vi "Save Station Information.vi"(8 "error in (no error)":errorcluster, 10 "Station Info":T1, 11 "TestMonitor in":refnum<class "TestMonitor.lvclass">) -> (0 "error out":errorcluster, 3 "TestMonitor out":refnum<class "TestMonitor.lvclass">)   [LabVIEW 2018, in "TestMonitor.lvclass"]
doc: "This VI will save the Station Information to the permanent report."
uses:
  TestMonitor.lvclass
  Report Information/Station Information.ctl
  TestMonitor.lvclass/TestMonitor.ctl
  <vilib>/Skyline/TestMonitor/Test Result/Update Test Result (Single).vi
  <vilib>/Skyline/TestMonitor/Test Result/NI SystemLink Test Result.lvclass
  Report Information/Report Information.lvclass
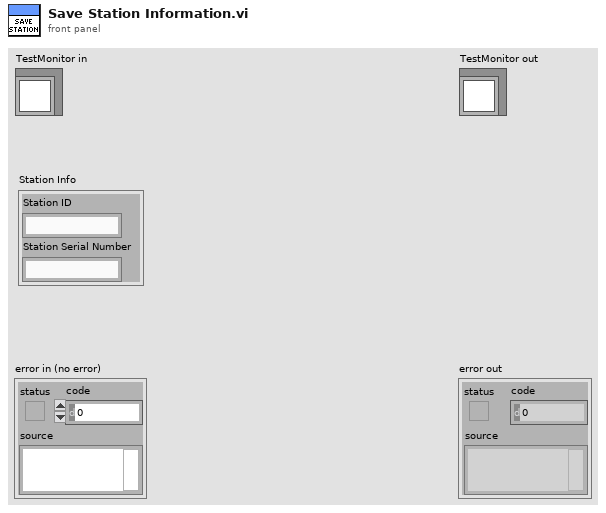
[diagram p1: front panel]
types:
  T1 = typedef "Report Information.lvclass/Station Information.ctl" = cluster{"Station ID":string, "Station Serial Number":string}
  T2 = typedef "NI Skyline Utilities.lvlib/Property.ctl" = cluster{"key":string, "value":string}
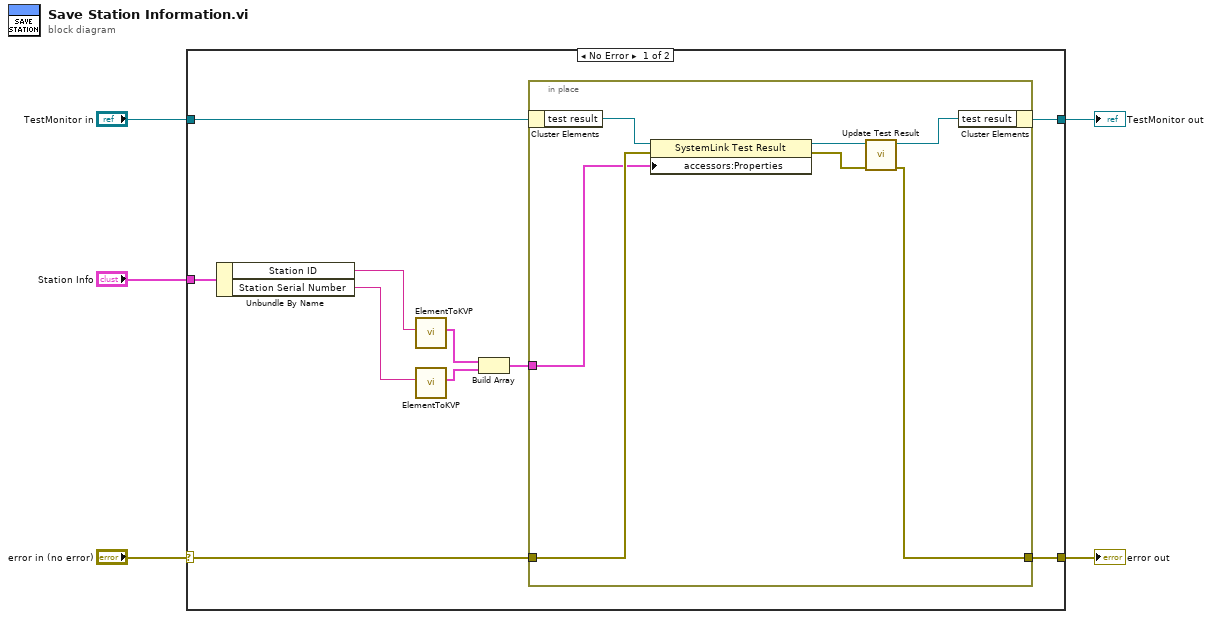
[diagram p0: block diagram]
diagram:
  n1 = case shown="No Error" "error in (no error)" {
    selector: "error in (no error)" -> [w12 w23]
    tunnel: [w10 w23] -> w5
    tunnel: [w14 w24] -> w3
    tunnel: "TestMonitor in" -> [w15 w24]
    tunnel: "Station Info" -> [w13 _]
    frame No Error {
      n2 = Unbundle By Name(w13) -> ("Station ID"=w9:string, "Station Serial Number"=w6:string)
      n3 = call "ElementToKVP.vi"("Element"=w9) -> ("KVP"=w8:T2)  [unwired: 9 in, 1 out]
      n4 = call "ElementToKVP.vi"("Element"=w6) -> ("KVP"=w7:T2)  [unwired: 9 in, 1 out]
      n5 = Build Array(w8, w7) -> (w11:T2[])
      n6 = in-place {
        in-place-border: w12 -> [w21]
        in-place-border: w11 -> [w20]
        in-place-border: [w16] -> w10
        n7 = in-place-cluster #1(w15) -> ("test result"=w22:refnum<class "NI SystemLink Test Result.lvclass">)
        n8 = property class="SystemLink Test Result"(reference=w22, error in=w21, "accessors:Properties"=w20) -> (reference out=w19:refnum<class "NI SystemLink Test Result.lvclass">, error out=w17:errorcluster)
        n9 = call-poly <vilib>:"Update Test Result.vi"("error in (no error)"=w17, "test result in"=w19) -> ("error out"=w16:errorcluster, "test result out"=w18:refnum<class "NI SystemLink Test Result.lvclass">)  [unwired: 8 in]
        n10 = in-place-cluster #1("test result"=w18) -> (w14:refnum<class "TestMonitor.lvclass">)
      }
    }
    frame Error {
    }
  }
  "error out" <- w5
  "TestMonitor out" <- w3
